vi "Read configuration.vi"(8 "error in (no error)":errorcluster, 11 "DIO Channel in":refnum<class "Digital IO Channel.lvclass">) -> (0 "error out":errorcluster, 2 "configuration":refnum<class "CEF_serializable configuration.lvclass">, 3 "DIO Channel out":refnum<class "Digital IO Channel.lvclass">)   [LabVIEW 2025, in "Digital IO.lvlib" / "Digital IO Channel.lvclass"]
uses:
  Digital IO Channel.lvclass
  Users/Public/Documents/Sandia National Labs/TSS Plugin/CEF.lvlibp/serializable configuration/CEF_serializable configuration.lvclass
  Digital IO Channel.lvclass/Digital IO Channel.ctl
  Digital IO Channel configuration/Digital IO Channel configuration.lvclass
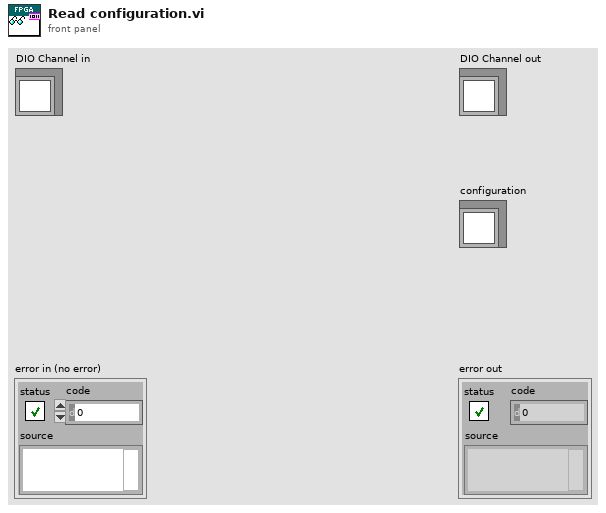
[diagram p1: front panel]
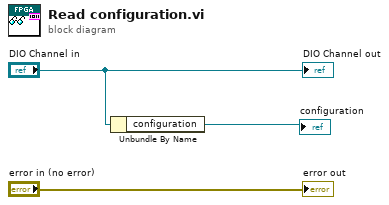
[diagram p0: block diagram]
diagram:
  n1 = Unbundle By Name("DIO Channel in") -> ("configuration"=→"configuration":refnum<class "Digital IO Channel configuration.lvclass">)
  "error out" <- "error in (no error)"
  "DIO Channel out" <- "DIO Channel in"
